vi "Write Fixture ID.vi"(8 "error in (no error)":errorcluster, 10 "Fixture ID":string[](array[string]), 11 "TestBench in":refnum<class "TestBench.lvclass">) -> (0 "error out":errorcluster, 3 "TestBench out":refnum<class "TestBench.lvclass">)   [LabVIEW 2019, in "TestBench.lvlib" / "TestBench.lvclass"]
uses:
  TestBench.lvclass
  TestBench.lvclass/TestBench.ctl
  LocalReport/LocalReport Messages/InitializeReport Msg/InitializeReport Msg.lvclass/InitializeReport Msg.ctl
  <vilib>/ActorFramework/Message Enqueuer/Message Enqueuer.lvclass/Message Enqueuer.ctl
  TestSetup/TestSetup Messages/Write TestLimitPath Msg/Write TestLimitPath Msg.lvclass/Write TestLimitPath Msg.ctl
  3a89b56f-d663-4f9e-9b9b-cc859f135345.vi
  5fc22ac5-6f4d-4095-becc-867abee3661b.vi
  987c4875-a7cd-4ca8-9df8-e4c83021dc58.vi
  <vilib>/ActorFramework/Message Enqueuer/Enqueue.vi
  LocalReport/LocalReport Messages/InitializeReport Msg/InitializeReport Msg.lvclass
  C:/Program Files (x86)/National Instruments/LabVIEW 2019/vi.lib/ActorFramework/Message/Message.lvclass
  TestSetup/TestSetup Messages/Write TestLimitPath Msg/Write TestLimitPath Msg.lvclass
  <vilib>/ActorFramework/Message Priority Queue/Priority Enqueue.vi
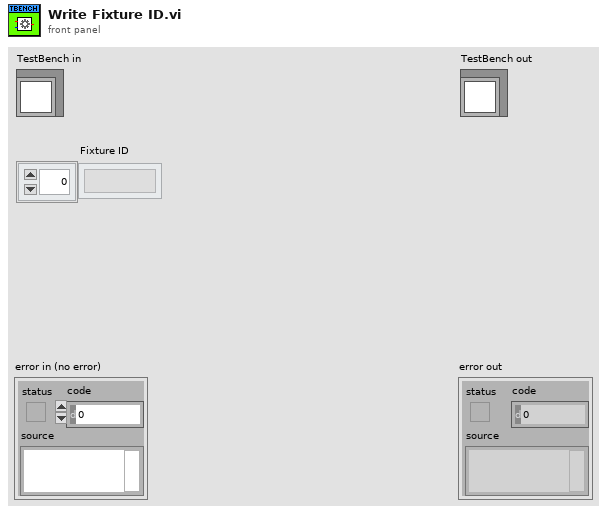
[diagram p1: front panel]
types:
  T1 = typedef "SoftwareSetup.lvlib/Local Report.ctl" = cluster{"Report Path":path, "Report  Format":enum16{"CSV", "XML", "PDF", "Excel", "TXT"}, "Disabled State":bool, "Customer name":string}
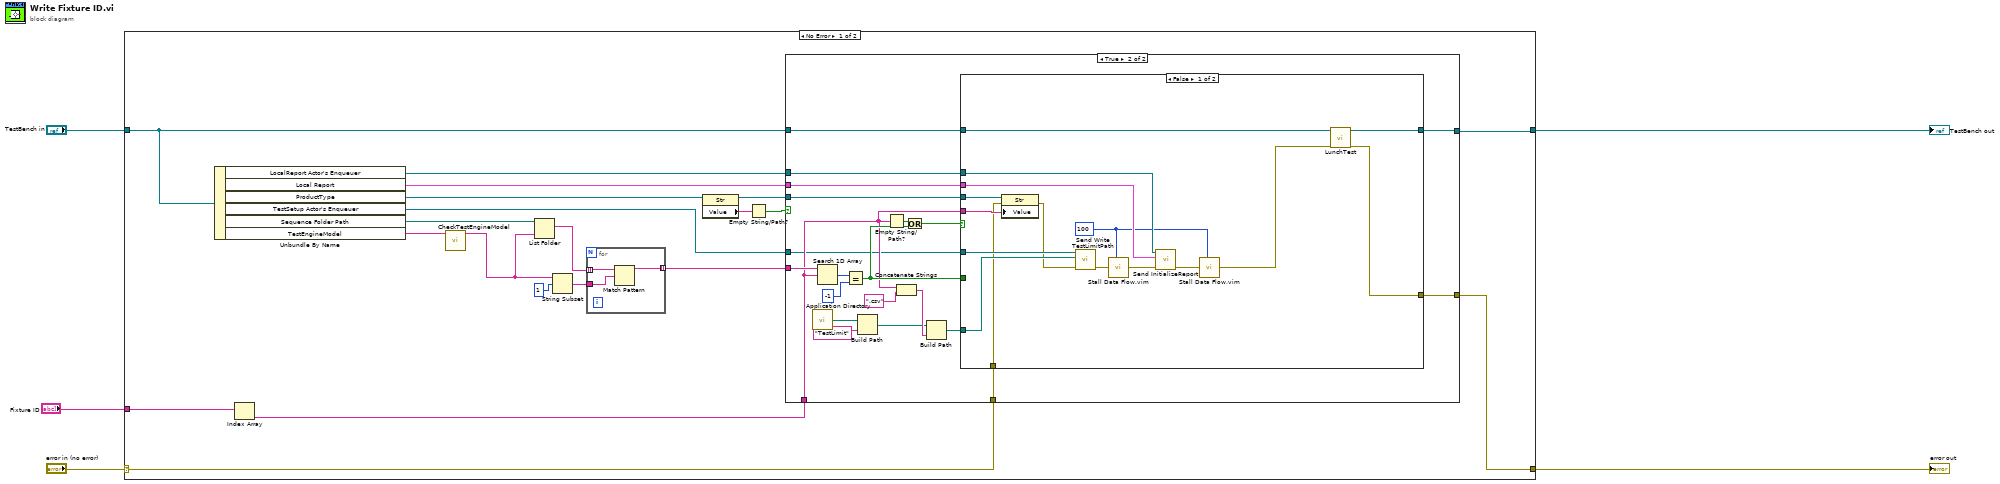
[diagram p0: block diagram]
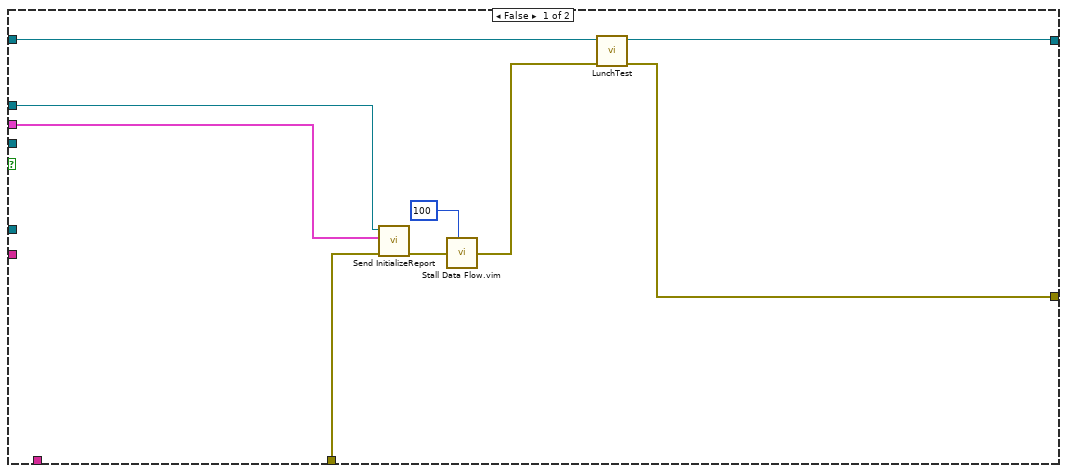
[diagram p2: hidden frame]
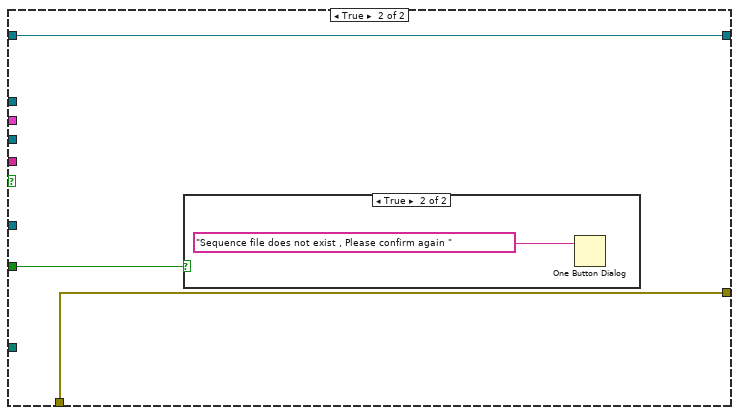
[diagram p3: hidden frame]
diagram:
  n1 = case shown="No Error" "error in (no error)" {
    selector: "error in (no error)" -> [w14 w79]
    tunnel: [w6 w79] -> w4
    tunnel: [w7 w80] -> w2
    tunnel: "TestBench in" -> [w11 w80]
    tunnel: "Fixture ID" -> [w19 _]
    frame No Error {
      n2 = Unbundle By Name(w11) -> ("LocalReport Actor's Enqueuer"=w13:refnum<class "Message Enqueuer.lvclass">, "Local Report"=w12:T1, "ProductType"=w15:refnum<vi>, "TestSetup Actor's Enqueuer"=w16:refnum<class "Message Enqueuer.lvclass">, "Sequence Folder Path"=w21:path, "TestEngineModel"=w20:string)
      n3 = Index Array(array=w19) -> (element=w17:string)  [unwired: 1 in]
      n4 = call "CheckTestEngineModel.vi"("Modle"=w20) -> ("Pattern"=w25:string)  [unwired: 10 in]
      n5 = List Folder(path=w21, pattern=w25) -> (filenames=w23:string[])  [unwired: 2 in, 3 out]
      n6 = String Subset(string=w25, offset (0)=1) -> (substring=w24:string)  [unwired: 1 in]
      n7 = for {
        tunnel: w23 -> [w78] mode=indexing
        tunnel: [w77] -> w18 mode=indexing
        tunnel: w24 -> [w76]
        n8 = Match Pattern(string=w78, regular expression=w76) -> (before substring=w77:string)  [unwired: 1 in, 3 out]
      }
      n9 = property class="Str"(reference=w15) -> (reference out=w10:refnum<vi>, "Value"=w9:string)  [unwired: 1 in, 1 out]
      n10 = Empty String/Path?(string/path=w9) -> (empty?=w8:bool)
      n11 = case shown="True" w8 {
        tunnel: w18 -> [_ w44]
        tunnel: w17 -> [_ w43]
        tunnel: w16 -> [_ w42]
        tunnel: w14 -> [w28 w41]
        tunnel: w13 -> [w31 w40]
        tunnel: w12 -> [w30 w39]
        tunnel: w11 -> [w32 w38]
        tunnel: w10 -> [_ w37]
        tunnel: [w27 w36] -> w7
        tunnel: [w26 w35] -> w6
        frame False {
          n12 = call "Send InitializeReport.vi"("error in (no error)"=w28, "Local Report Parameter"=w30, "Message Enqueuer"=w31) -> ("error out"=w34:errorcluster)  [unwired: 7 in, 1 out]
          n13 = call "Stall Data Flow.vim"("value in"=w34, "milliseconds to wait"=u32 100) -> ("value out"=w33:errorcluster)  [unwired: 1 out]
          n14 = call-dynamic "LunchTest.vi"("error in (no error)"=w33, "TestBench in"=w32) -> ("error out"=w26:errorcluster, "TestBench out"=w27:refnum<class "TestBench.lvclass">)  [unwired: 8 in]
        }
        frame True {
          n15 = call <vilib>:"Application Directory.vi"() -> ("Application Directory"=w53:path)
          n16 = Search 1D Array(1D array=w44, element=w43) -> (index of element=w48:i32)  [unwired: 1 in]
          n17 = Equal?(x=w48, y=-1) -> (x = y?=w45:bool)
          n18 = Build Path(base path=w53, name or relative path="TestLimit") -> (appended path=w50:path)
          n19 = Empty String/Path?(string/path=w43) -> (empty?=w55:bool)
          n20 = Concatenate Strings(w43, ".csv" ("string")) -> (w51:string)
          n21 = Or(x=w55, y=w45) -> (x .or. y?=w46:bool)
          n22 = Build Path(base path=w50, name or relative path=w51) -> (appended path=w49:path)
          n23 = case shown="False" w46 {
            tunnel: w37 -> [w71 _]
            tunnel: w43 -> [w70 _]
            tunnel: w49 -> [w68 _]
            tunnel: w42 -> [w69 _]
            tunnel: w45 -> [_ w74]
            tunnel: [w60 w73] -> w35
            tunnel: w41 -> [w66 w73]
            tunnel: w40 -> [w58 _]
            tunnel: w39 -> [w59 _]
            tunnel: w38 -> [w62 w72]
            tunnel: [w61 w72] -> w36
            frame False {
              w56 = u32 100 ("milliseconds to wait")
              n24 = property class="Str"(reference=w71, error in=w66, "Value"=w70) -> (error out=w67:errorcluster)  [unwired: 1 out]
              n25 = call "Send Write TestLimitPath.vi"("error in (no error)"=w67, "TestLimitPath"=w68, "Message Enqueuer"=w69) -> ("error out"=w63:errorcluster)  [unwired: 7 in, 1 out]
              n26 = call "Stall Data Flow.vim"("value in"=w63, "milliseconds to wait"=w56) -> ("value out"=w57:errorcluster)  [unwired: 1 out]
              n27 = call "Send InitializeReport.vi"("error in (no error)"=w57, "Local Report Parameter"=w59, "Message Enqueuer"=w58) -> ("error out"=w65:errorcluster)  [unwired: 7 in, 1 out]
              n28 = call "Stall Data Flow.vim"("value in"=w65, "milliseconds to wait"=w56) -> ("value out"=w64:errorcluster)  [unwired: 1 out]
              n29 = call-dynamic "LunchTest.vi"("error in (no error)"=w64, "TestBench in"=w62) -> ("error out"=w60:errorcluster, "TestBench out"=w61:refnum<class "TestBench.lvclass">)  [unwired: 8 in]
            }
            frame True {
              n30 = case shown="True" w74 {
                frame False {
                }
                frame True {
                  n31 = One Button Dialog(message="Sequence file does not exist , Please confirm again ") -> ()  [unwired: 1 in, 1 out]
                }
              }
            }
          }
        }
      }
    }
    frame Error {
    }
  }
  "error out" <- w4
  "TestBench out" <- w2
